vi "FindUSBDevice.vi"(11 "DevSNin":string) -> (0 "DevSN":string, 1 "BOARD_INFO":T1, 2 "DevNum":i32=-1, 3 "Total":u32, 5 "SNs":string[](array[string]))   [LabVIEW 2011]
uses:
  data/ControlCAN.dll
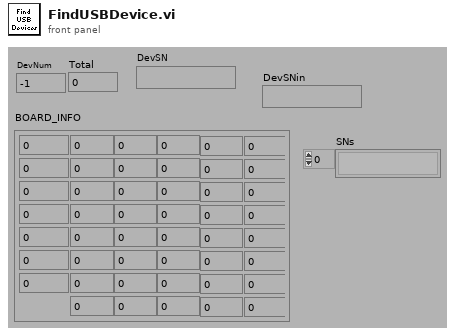
[diagram p1: front panel]
types:
  T1 = cluster{"hw_Version":u16, "fw_Version":u16, "dr_Version":u16, "in_Version":u16, "irq_Num":u16, "can_Num":u8, "reserved":u8, "sSN0":u8, "sSN1":u8, "sSN2":u8, "sSN3":u8, "sSN4":u8, "sSN5":u8, "sSN6":u8, "sSN7":u8, "shwT0":u8, "shwT1":u8, "shwT2":u8, "shwT3":u8, "shwT4":u8, "shwT5":u8, "shwT6":u8, "shwT7":u8, "shwT8":u8, "shwT9":u8, "shwT10":u8, "shwT11":u8, "shwT12":u8, "shwT13":u8, "shwT14":u8, "shwT15":u8, "sUSN0":u8, "sUSN1":u8, "sUSN2":u8, "sUSN3":u8, "sUSN4":u8, "sUSN5":u8, "sUSN6":u8, "sUSN7":u8, "sUSN8":u8, "sUSN9":u8, "sUSN10":u8, "sUSN11":u8, "sUSN12":u8, "sUSN13":u8, "sUSN14":u8, "sUSN15":u8}
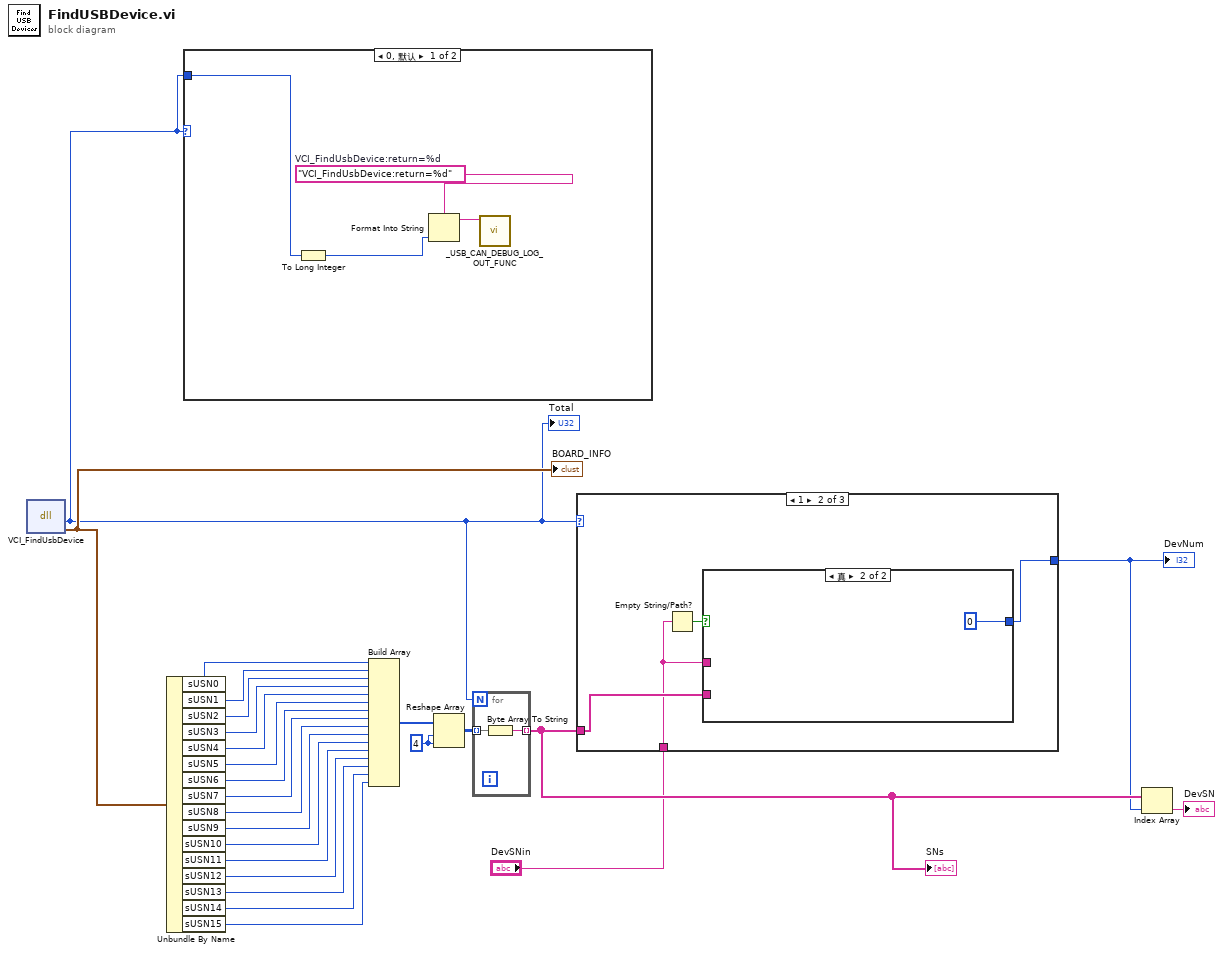
[diagram p0: block diagram]
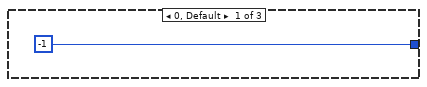
[diagram p3: hidden frame]
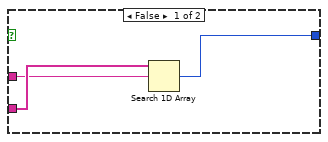
[diagram p4: hidden frame]
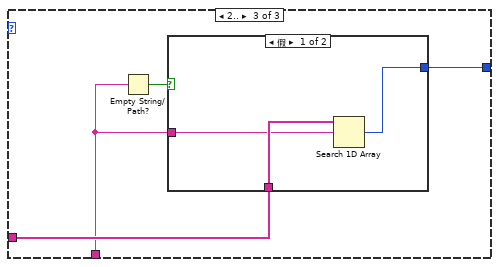
[diagram p5: hidden frame]
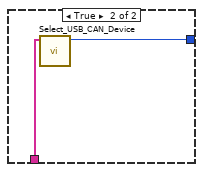
[diagram p6: hidden frame]
diagram:
  w24 = 4 ("维数大小")
  n1 = dll-call lib="PTH1Mabs ZHost_E工作TnewcodeUSB CAN Tool1.97dataControlCAN.dll" fn="VCI_FindUsbDevice"() -> ("返回类型"=w1:u32, "BOARD_INFO"=w6:T1)  [unwired: 4 in, 2 out]
  "Total" <- w1
  "BOARD_INFO" <- w6
  n2 = Unbundle By Name(w6) -> ("sUSN0"=w7:u8, "sUSN1"=w8:u8, "sUSN2"=w9:u8, "sUSN3"=w10:u8, "sUSN4"=w11:u8, "sUSN5"=w12:u8, "sUSN6"=w13:u8, "sUSN7"=w14:u8, "sUSN8"=w15:u8, "sUSN9"=w16:u8, "sUSN10"=w17:u8, "sUSN11"=w18:u8, "sUSN12"=w19:u8, "sUSN13"=w20:u8, "sUSN14"=w21:u8, "sUSN15"=w22:u8)
  n3 = case shown="0, 默认" w1 {
    tunnel: w1 -> [w28 _]
    frame 0, Default {
      w27 = "VCI_FindUsbDevice:return=%d"  # VCI_FindUsbDevice:return=%d
      n4 = To Long Integer(number=w28) -> (32bit integer=w26:i32)
      n5 = Format Into String(format string=w27, w26) -> (resulting string=w29:string)  [unwired: 2 in, 1 out]
      n6 = call "_USB_CAN_DEBUG_LOG_OUT_FUNC.vi"("Info"=w29) -> ()  [unwired: 11 in]
    }
    frame 1.. {
    }
  }
  n7 = Build Array(w7, w8, w9, w10, w11, w12, w13, w14, w15, w16, w17, w18, w19, w20, w21, w22) -> (w23:u8[])
  n8 = Reshape Array(w23, w24, w24) -> (w25:u8[][])
  n9 = for {
    N: w1 -> [_]
    tunnel: w25 -> [w31] mode=indexing
    tunnel: [w30] -> w5 mode=indexing
    n10 = Byte Array To String(unsigned byte array=w31) -> (string=w30:string)
  }
  "SNs" <- w5
  n11 = case shown="1" w1 {
    tunnel: [-1 ("DevNum") w35 w44] -> w2
    tunnel: w5 -> [_ w34 w43]
    tunnel: "DevSNin" -> [_ w33 w41]
    frame 0, Default {
    }
    frame 1 {
      n12 = Empty String/Path?(string/path=w33) -> (empty?=w36:bool)
      n13 = case shown="真" w36 {
        tunnel: [w37 0 ("DevNum")] -> w35
        tunnel: w34 -> [w39 _]
        tunnel: w33 -> [w38 _]
        frame False {
          n14 = Search 1D Array(1D array=w39, element=w38) -> (index of element=w37:i32)  [unwired: 1 in]
        }
        frame True {
        }
      }
    }
    frame 2.. {
      n15 = Empty String/Path?(string/path=w41) -> (empty?=w42:bool)
      n16 = case shown="假" w42 {
        tunnel: [w45 w49] -> w44
        tunnel: w43 -> [w47 w48]
        tunnel: w41 -> [w46 _]
        frame False {
          n17 = Search 1D Array(1D array=w47, element=w46) -> (index of element=w45:i32)  [unwired: 1 in]
        }
        frame True {
          n18 = call "Select_USB_CAN_Device.vi"("DevNames"=w48) -> ("DevNum"=w49:i32)  [unwired: 10 in]
        }
      }
    }
  }
  "DevNum" <- w2
  n19 = Index Array(array=w5, index=w2) -> (element=→"DevSN":string)
